vi "Save All VI Data.vi"(8 "error in (no error)":errorcluster, 11 "VI Data":T1[](array[typedef])) -> (0 "error out":errorcluster, 3 "VI Data out":T1[](array[typedef]))   [LabVIEW 2023, in "VI Properties Editor.lvlib"]
uses:
  VI Properties Editor.lvlib
  Cluster Data.ctl
  <vilib>/picture/picture.llb/imagedata.ctl
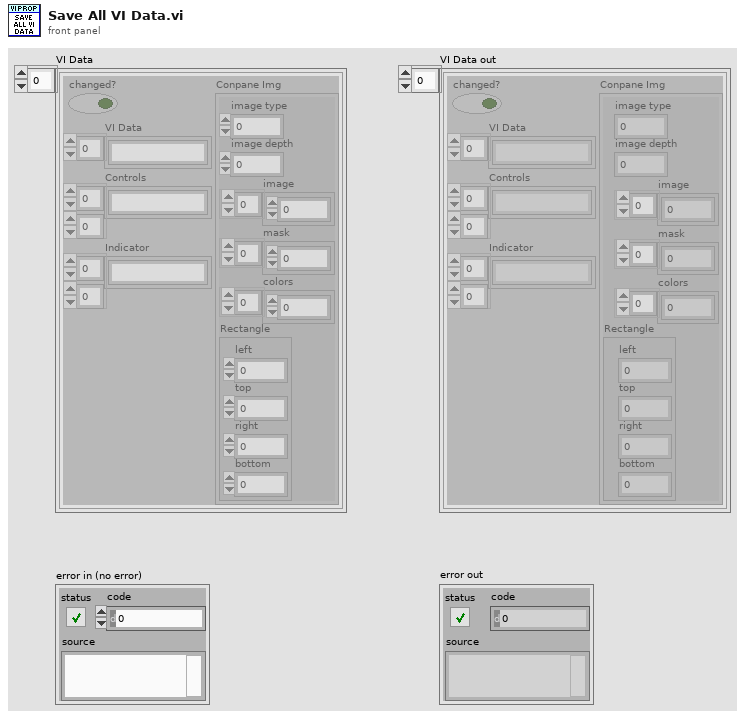
[diagram p1: front panel]
types:
  T1 = typedef "VI Properties Editor.lvlib/Cluster Data.ctl" = cluster{"changed?":bool, "VI Data":string[], "Controls":string[][], "Indicator":string[][], "Conpane Img":T2}
  T2 = typedef "imagedata.ctl" = cluster{"image type":i32, "image depth":i32, "image":u8[], "mask":u8[], "colors":u32[], "Rectangle":cluster{"left":i16, "top":i16, "right":i16, "bottom":i16}}
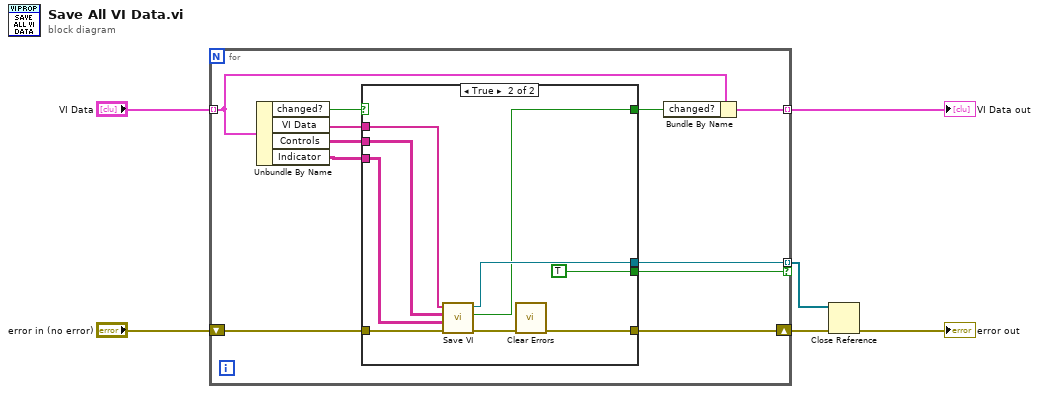
[diagram p0: block diagram]
diagram:
  n1 = for {
    shift-right: [w15] -> w3
    shift-left: "error in (no error)" -> [w17]
    tunnel: "VI Data" -> [w12] mode=indexing
    tunnel: [w16] -> w2 mode=indexing if=w14
    tunnel: [w10] -> w5 mode=indexing
    n2 = Unbundle By Name(w12) -> ("changed?"=w13:bool, "VI Data"=w9:string[], "Controls"=w8:string[][], "Indicator"=w7:string[][])
    n3 = case shown="True" w13 {
      selector: w13 -> [w18 _]
      tunnel: w9 -> [_ w30]
      tunnel: w17 -> [w20 w29]
      tunnel: [refnum<k0> refnum w28] -> w16
      tunnel: [w20 w27] -> w15
      tunnel: [FALSE TRUE] -> w14
      tunnel: [w18 w24] -> w11
      tunnel: w8 -> [_ w23]
      tunnel: w7 -> [_ w22]
      frame False {
      }
      frame True {
        n4 = call "Save VI.vi"("error in (no error)"=w29, "Indicator"=w22, "Controls"=w23, "Data"=w30) -> ("error out"=w25:errorcluster, "status"=w24:bool, "VI out"=w28:refnum<vi>)  [unwired: 5 in]
        n5 = call <vilib>:"Clear Errors.vi"("error in (no error)"=w25) -> ("error out"=w27:errorcluster)  [unwired: 5 in, 1 out]
      }
    }
    n6 = Bundle By Name(cluster=w12, "changed?"=w11) -> (w10:T1)
  }
  "VI Data out" <- w5
  n7 = Close Reference(reference=w2, error in (no error)=w3) -> (error out=→"error out":errorcluster)
